vi "Write RingdownConfig.vi"(8 "error in (no error)":errorcluster, 10 "RingdownConfig":T1={"Config"={"p_SysOdr"=-1, "dThres"=0.0, "Preproc"={"order"=0, "f_lo"=1000.0, "f_hi"=1000.0, "R_down"=-1}}, "V index"=0, "I index"=3, "PosSeq"=FALSE}, 11 "RingdownPlugin in":refnum<class "EraPlugin.lvclass">) -> (0 "error out":errorcluster, 3 "RingdownPlugin out":refnum<class "EraPlugin.lvclass">)   [LabVIEW 2017, in "AppPlugins.lvlib" / "ERAPlugin.lvclass"]
uses:
  EraPlugin.lvclass
  PublicAPI/TypeDef/RingdownConfig.ctl
  EraPlugin.lvclass/EraPlugin.ctl
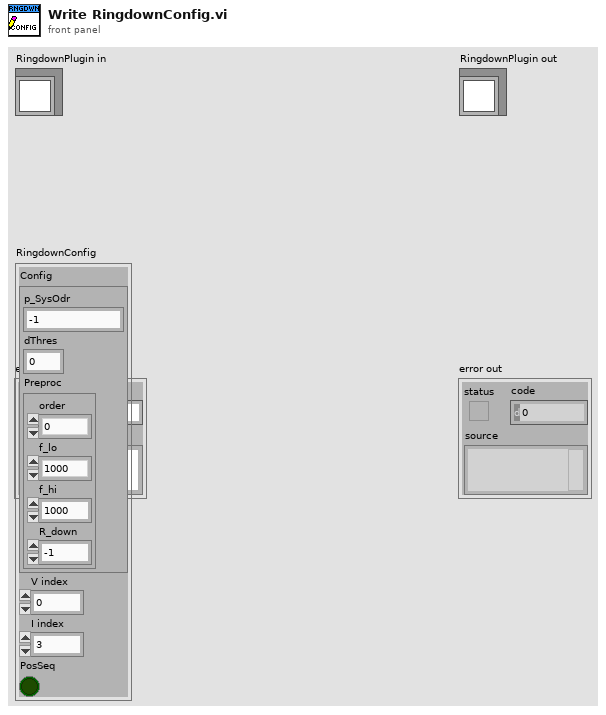
[diagram p1: front panel]
types:
  T1 = typedef "AppPlugins.lvlib/ERAPlugin.lvclass/RingdownConfig.ctl" = cluster{"Config":cluster{"p_SysOdr":i32, "dThres":dbl, "Preproc":cluster{"order":i32, "f_lo":dbl, "f_hi":dbl, "R_down":i32}}, "V index":i32, "I index":i32, "PosSeq":bool}
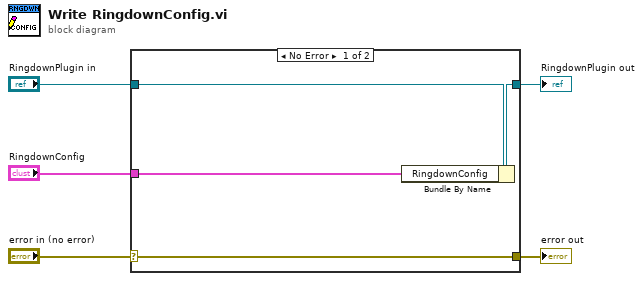
[diagram p0: block diagram]
diagram:
  n1 = case shown="No Error" "error in (no error)" {
    selector: "error in (no error)" -> [w9 w10]
    tunnel: [w9 w10] -> w4
    tunnel: [w7 w11] -> w2
    tunnel: "RingdownPlugin in" -> [w8 w11]
    tunnel: "RingdownConfig" -> [w6 _]
    frame No Error {
      n2 = Bundle By Name(cluster=w8, "RingdownConfig"=w6) -> (w7:refnum<class "EraPlugin.lvclass">)
    }
    frame Error {
    }
  }
  "error out" <- w4
  "RingdownPlugin out" <- w2
